vi "deltaPS.vi"(8 "error in (no error)":errorcluster, 11 "VISA Refnum in":refnum<visa-resource-name>) -> (0 "error out":errorcluster, 3 "DeltaPS":string)   [LabVIEW 2019]
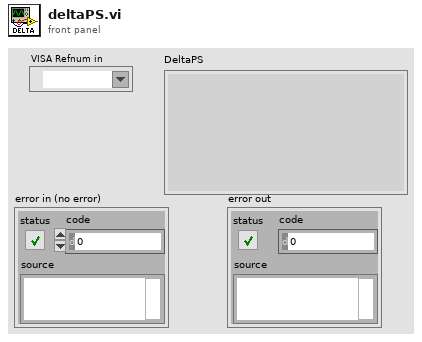
[diagram p1: front panel]
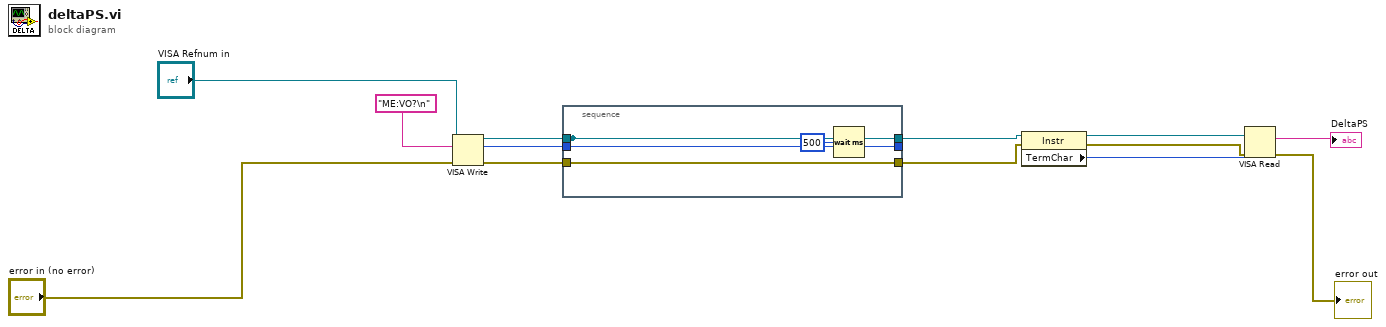
[diagram p0: block diagram]
diagram:
  n1 = VISA Write(VISA resource name="VISA Refnum in", write buffer="ME:VO?\n", error in (no error)="error in (no error)") -> (VISA resource name out=w10:refnum<visa-resource-name>, return count=w8:u32, error out=w9:errorcluster)
  n2 = stacked-sequence {
    tunnel: [w16] -> _
    tunnel: w10 -> [w16]
    tunnel: w9 -> [w14]
    tunnel: w8 -> [w15]
    tunnel: [w16] -> w7
    tunnel: [w15] -> _
    tunnel: [w14] -> w6
    frame #0 {
      n3 = Wait (ms)(milliseconds to wait=u32 500) -> ()  [unwired: 1 out]
    }
  }
  n4 = property class="Instr"(reference=w7, error in=w6) -> (reference out=w5:refnum<visa-resource-name>, error out=w4:errorcluster, "TermChar"=w3:u8)
  n5 = VISA Read(VISA resource name=w5, byte count=w3, error in (no error)=w4) -> (read buffer=→"DeltaPS":string, error out=→"error out":errorcluster)  [unwired: 2 out]
